vi "Calculate Wall Lines Size.vi"(10 "Brick Wall":T1[](array[typedef]), 11 "Y Size":i32) -> (3 "Lines Size List":i32[](array[numeric]))   [LabVIEW 2017]
uses:
  Controls/Coordinates.ctl
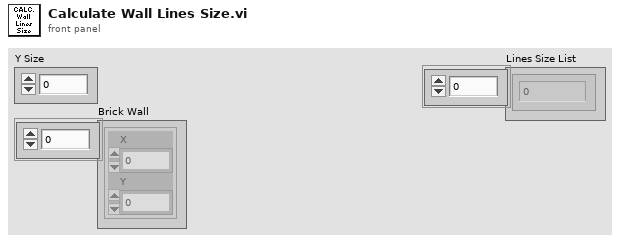
[diagram p1: front panel]
types:
  T1 = typedef "Coordinates.ctl" = cluster{"X":i32, "Y":i32}
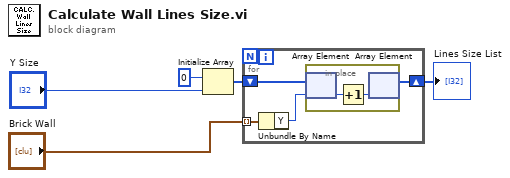
[diagram p0: block diagram]
diagram:
  n1 = Initialize Array(0, "Y Size") -> (w3:i32[])
  n2 = for {
    tunnel: "Brick Wall" -> [w9] mode=indexing
    shift-right: [w7] -> w1
    shift-left: w3 -> [w8]
    n3 = Unbundle By Name(w9) -> ("Y"=w6:i32)
    n4 = in-place {
      n5 = in-place-array #1(w8, w6) -> (w11:i32)
      n6 = Increment(x=w11) -> (x+1=w10:i32)
      n7 = in-place-array #1(w10) -> (w7:i32[])  [unwired: 1 out]
    }
  }
  "Lines Size List" <- w1
